vi "Test Set Subpanels.vi"(8 "error in":errorcluster) -> (0 "error out":errorcluster)   [LabVIEW 2019]
uses:
  <vilib>/addons/_JKI Toolkits/Caraya/classes/Test/Test.lvclass
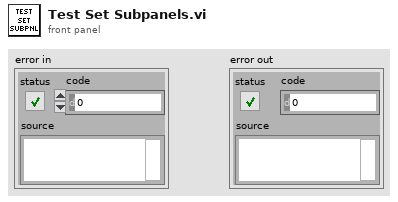
[diagram p1: front panel]
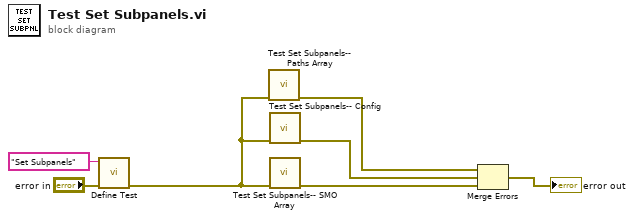
[diagram p0: block diagram]
diagram:
  n1 = call <vilib>:"Define Test.vi"("error in (no error)"="error in", "Label (VI Title)"="Set Subpanels") -> ("error out"=w2:errorcluster)  [unwired: 9 in]
  n2 = call "Test Set Subpanels-- Paths Array.vi"("error in"=w2) -> ("error out"=w1:errorcluster)  [unwired: 10 in]
  n3 = call "Test Set Subpanels-- Config.vi"("error in"=w2) -> ("error out"=w3:errorcluster)  [unwired: 10 in]
  n4 = call "Test Set Subpanels-- SMO Array.vi"("error in"=w2) -> ("error out"=w4:errorcluster)  [unwired: 10 in]
  n5 = Merge Errors(w1, w3, w4) -> (→"error out":errorcluster)
